vi "mqttTCPIPInterpretFixedHeaderResponse.vi"(0 "data in":string, 11 "error in (no error)":errorcluster) -> (6 "remainingLengthByte1":u8, 8 "output cluster":T1={"retain"=FALSE, "qos"=enum."At most once", "duplicate"=FALSE, "response"=enum."CONNECT"}, 15 "error out":errorcluster)   [LabVIEW 2018, in "mqtt.lvclass"]
uses:
  mqtt.lvclass
  mqttTypedef/mqttFixedHeaderResponse.ctl
  mqttTypedef/mqttQOSlevel.ctl
  mqttTypedef/mqttMessageType.ctl
panel:
  out "rxTelegram (HEX)":u8[](array[numeric]) format="%x"
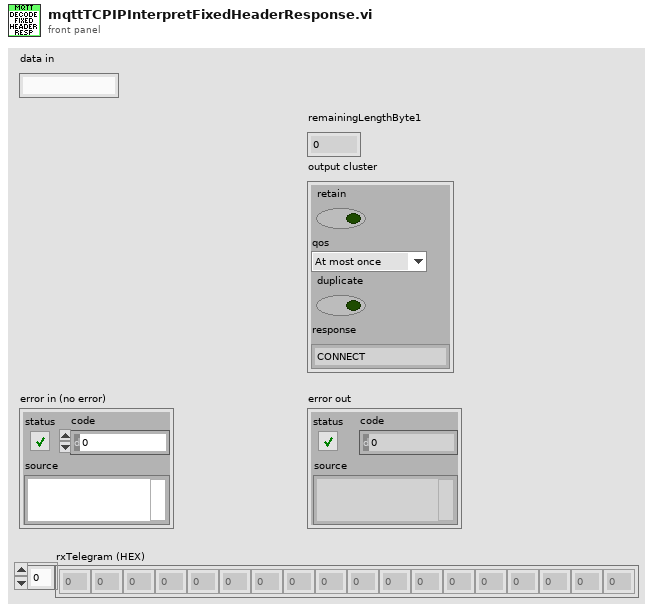
[diagram p1: front panel]
types:
  T1 = typedef "mqttFixedHeaderResponse.ctl" = cluster{"retain":bool, "qos":T2, "duplicate":bool, "response":T3}
  T2 = typedef "mqttQOSlevel.ctl" = enum8{"At most once", "At least once", "Exactly once", "Reserved"}
  T3 = typedef "mqttMessageType.ctl" = enum32{"Reserved", "CONNECT", "CONNACK", "PUBLISH", "PUBACK", "PUBREC", "PUBREL", "PUBCOMP", "SUBSCRIBE", "SUBACK", "UNSUBSCRIBE", "UNSUBACK", "PINGREQ", "PINGRESP", "DISCONNECT", "Reserved2"}
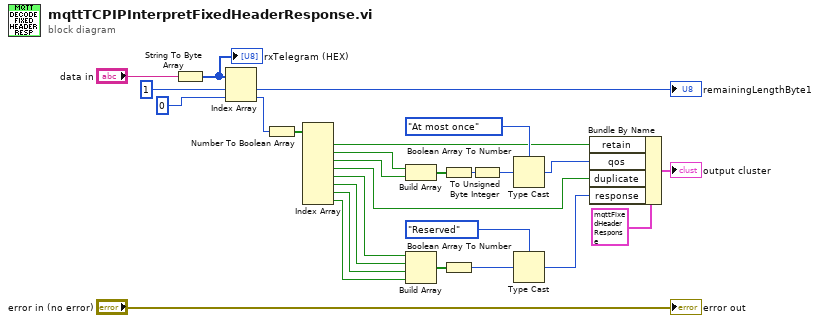
[diagram p0: block diagram]
diagram:
  n1 = String To Byte Array(string="data in") -> (unsigned byte array=w10:u8[])
  "rxTelegram (HEX)" <- w10
  n2 = Index Array(array=w10, index #1=1 ("index"), index #2=0 ("index")) -> (element #1=→"remainingLengthByte1":u8, element #2=w27:u8)
  n3 = Number To Boolean Array(number=w27) -> (Boolean array=w26:bool[])
  n4 = Index Array(array=w26) -> (element #1=w6:bool, element #2=w22:bool, element #3=w21:bool, element #4=w4:bool, element #5=w17:bool, element #6=w16:bool, element #7=w15:bool, element #8=w14:bool)  [unwired: 8 in]
  n5 = Build Array(w22, w21) -> (w23:bool[])
  n6 = Build Array(w17, w16, w15, w14) -> (w18:bool[])
  n7 = Boolean Array To Number(Boolean array=w23) -> (number=w24:u32)
  n8 = Boolean Array To Number(Boolean array=w18) -> (number=w19:u32)
  n9 = To Unsigned Byte Integer(number=w24) -> (unsigned 8bit integer=w25:u8)
  n10 = Type Cast(type=mqttQOSlevel."At most once" ("QoS"), x=w25) -> (*(type *) &x=w5:T2)
  n11 = Type Cast(type=mqttMessageType."Reserved" ("MessageType"), x=w19) -> (*(type *) &x=w3:T3)
  n12 = Bundle By Name(cluster=T1 {"retain"=FALSE, "qos"=enum."At most once", "duplicate"=FALSE, "response"=enum."CONNECT"}, "retain"=w6, "qos"=w5, "duplicate"=w4, "response"=w3) -> (→"output cluster":T1)
  "error out" <- "error in (no error)"
